vi "main_ctrl.vi"(8 "error in":errorcluster) -> (0 "error out":errorcluster caption="error")   [LabVIEW 2013]
uses:
  <vilib>/Rock Robotics/WPI/DriverStation/WPI_DriverStationRobotMode2.ctl
  typedefs/fg_typedef.ctl
  typedefs/vision enable.ctl
  typedefs/vision data.ctl
  typedefs/subStates.ctl
  typedefs/singleUseSubstate.ctl
  <vilib>/Rock Robotics/WPI/Solenoid/WPI_SolenoidValue.ctl
  <vilib>/Rock Robotics/WPI/Compressor/WPI_CompressorGetSetRefNum.vi
  <vilib>/Rock Robotics/WPI/RobotDrive/WPI_RobotDriveGetSetRefNum.vi
  <vilib>/Rock Robotics/WPI/RobotDrive/WPI_RobotDriveArcadeDrive_Standard(NoSaturation).vi
  <vilib>/Rock Robotics/WPI/Solenoid/WPI_SolenoidSetEnum.vi
panel:
  out "Robot Mode":T1
  out "Vision SPI":u32
  out "Vision IPS":dbl
  out "Main IPS":dbl
  out "Main SPI":u32
  # "MAIN CONTROL"
  # "holds robot control code - dual parallel state machine"
  # "SPI: milliseconds per iteration\nIPS: iterations per second"
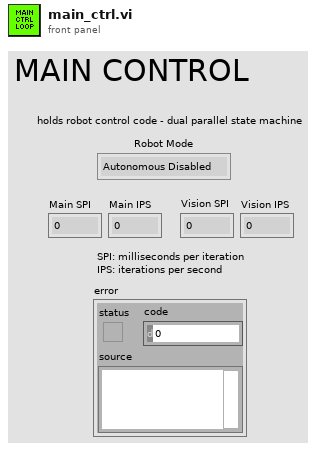
[diagram p1: front panel]
types:
  T1 = typedef "WPI_DriverStationRobotMode2.ctl" = enum16{"Autonomous Disabled", "Autonomous Enabled", "Teleop Disabled", "Teleop Enabled", "Timeout", "Finish", "Test Disabled", "Test Enabled"}
  T2 = typedef "vision data.ctl" = cluster{"x":dbl, "y":dbl, "area":dbl, "width":dbl, "height":dbl, "Hot Goal Present?":bool, "distance":dbl}
  T3 = typedef "vision enable.ctl" = enum16{"Enable", "Disable", "Stop"}
  T4 = typedef "fg_typedef.ctl" = enum16{"Get", "Set"}
  T5 = typedef "WPI_RobotDriveDevRef.ctl" = cluster{"DevStatus":errorcluster, "Motors[]":T6[], "Square Inputs":bool, "Max Output":dbl, "Isochronous":bool}
  T6 = typedef "WPI_MotorControlDeviceRef.ctl" = cluster{"DeviceStatus":errorcluster, "Type":enum16{"PWM", "CAN"}, "PWM":cluster{"Digital Module":T7, "PWM Channel":T8, "DeadBand":T9}, "CAN":cluster{"Device Number":u8, "Control Mode":T10, "Semaphore":T11, "Max Vout":dbl}, "Invert":bool, "TransformRef":T12, "InvTransformRef":T12}
  T7 = typedef "FPGA_TypedefDigitalModule.ctl" = enum16{"Digital Module 1", "Digital Module 2"}
  T8 = typedef "FPGA_DIOPWMChannel.ctl" = enum8{"PWM 1", "PWM 2", "PWM 3", "PWM 4", "PWM 5", "PWM 6", "PWM 7", "PWM 8", "PWM 9", "PWM 10", "Invalid"}
  T9 = typedef "WPI_PWMDeadband.ctl" = cluster{"Name":string, "maxPositivePwm":i32, "minPositivePwm":i32, "centerPwm":i32, "maxNegativePwm":i32, "minNegativePwm":i32, "angularRange":u16}
  T10 = typedef "WPI_CANJaguar_ControlMode.ctl" = enum8{"Percent VBus", "Current", "Speed", "Position", "Voltage"}
  T11 = typedef "Semaphore RefNum" = refnum<k1>
  T12 = typedef "WPI_PWMTransform_ConPane.ctl" = refnum<vi>
  T13 = typedef "WPI_CompressorDevRef.ctl" = cluster{"DevStatus":errorcluster, "DigitalInputDevRef":T14, "RelayDevRef":T16}
  T14 = typedef "WPI_DigitalInputDevRef.ctl" = cluster{"DevStatus":errorcluster, "DIO Channel":T15, "Digital Module":T7}
  T15 = typedef "FPGA_DIOChannel.ctl" = enum8{"DIO 1", "DIO 2", "DIO 3", "DIO 4", "DIO 5", "DIO 6", "DIO 7", "DIO 8", "DIO 9", "DIO 10", "DIO 11", "DIO 12", "DIO 13", "DIO 14", "Invalid"}
  T16 = typedef "WPI_RelayDevRef.ctl" = cluster{"DevStatus":errorcluster, "Relay Channel":T17, "Digital Module":T7, "Relay Direction":T18}
  T17 = typedef "FPGA_DIORelayChannel.ctl" = enum8{"Relay 1", "Relay 2", "Relay 3", "Relay 4", "Relay 5", "Relay 6", "Relay 7", "Relay 8", "Invalid"}
  T18 = typedef "WPI_RelayDirection.ctl" = enum16{"Both directions", "Forward only", "Reverse only"}
  T19 = typedef "WPI_CameraDevRef.ctl" = cluster{"Camera Address":string, "CameraStatus":errorcluster, "Acquire Image Notifier":refnum<notifier>}
  T20 = typedef "WPI_SolenoidDevRef.ctl" = cluster{"DevStatus":errorcluster, "Solenoid Module":T21, "Forward Solenoid Channel":T22, "Reverse Solenoid Channel":T22}
  T21 = typedef "FPGA_TypedefSolenoidModule.ctl" = enum16{"Solenoid Module 1", "Solenoid Module 2"}
  T22 = typedef "WPI_SolenoidChannel.ctl" = enum8{"Solenoid 1", "Solenoid 2", "Solenoid 3", "Solenoid 4", "Solenoid 5", "Solenoid 6", "Solenoid 7", "Solenoid 8", "Invalid"}
  T23 = typedef "IMAQ Image.ctl" = refnum<image>
  T24 = typedef "WPI_SolenoidValue.ctl" = enum16{"Off", "On", "Forward", "Reverse"}
  T25 = typedef "singleUseSubstate.ctl" = enum16{"null", "wait", "shift high", "shift low"}
  T26 = typedef "WPI_DriverStationDerivedRobotMode.ctl" = enum16{"Init", "Execute", "Stop"}
  T27 = typedef "subStates.ctl" = enum16{"null", "wait", "driver control", "auto", "manual override", "hold position", "rotate", "pickup", "pass", "load", "cock", "goto shoot", "shoot", "end"}
  T28 = typedef "Loop 2 Datatype.ctl" = cluster{"State":T27, "Waiting Loop":i32, "State to Wait For":i32, "Loop ID":i32, "Exit Value":i32, "Joystick":dbl}
  T29 = typedef "Loop 1 Datatype.ctl" = cluster{"State":T27, "Waiting Loop":i32, "State to Wait For":i32, "Loop ID":i32, "Exit Value":i32, "Joystick":dbl, "Index Up":bool, "Index Down":bool}
  T30 = typedef "Loop 3 Datatype.ctl" = cluster{"State":T27, "Waiting Loop":i32, "State to Wait For":i32, "Loop ID":i32, "Exit Value":i32, "Joystick":dbl, "Z Axis":dbl}
  T31 = typedef "Loop 0 Datatype.ctl" = cluster{"State":T27, "Waiting Loop":i32, "State to Wait For":i32, "Loop ID":i32, "Exit Value":i32, "X Axis":dbl, "Y Axis":dbl, "Z Axis":dbl}
  T32 = typedef "Loop 4 Datatype.ctl" = cluster{"State":T27, "Waiting Loop":i32, "State to Wait For":i32, "Loop ID":i32, "Exit Value":i32, "Joystick":dbl}
  T33 = cluster{"Vision mSPI":u32, "Main mSPI":u32, "Dash mSPI":u32}
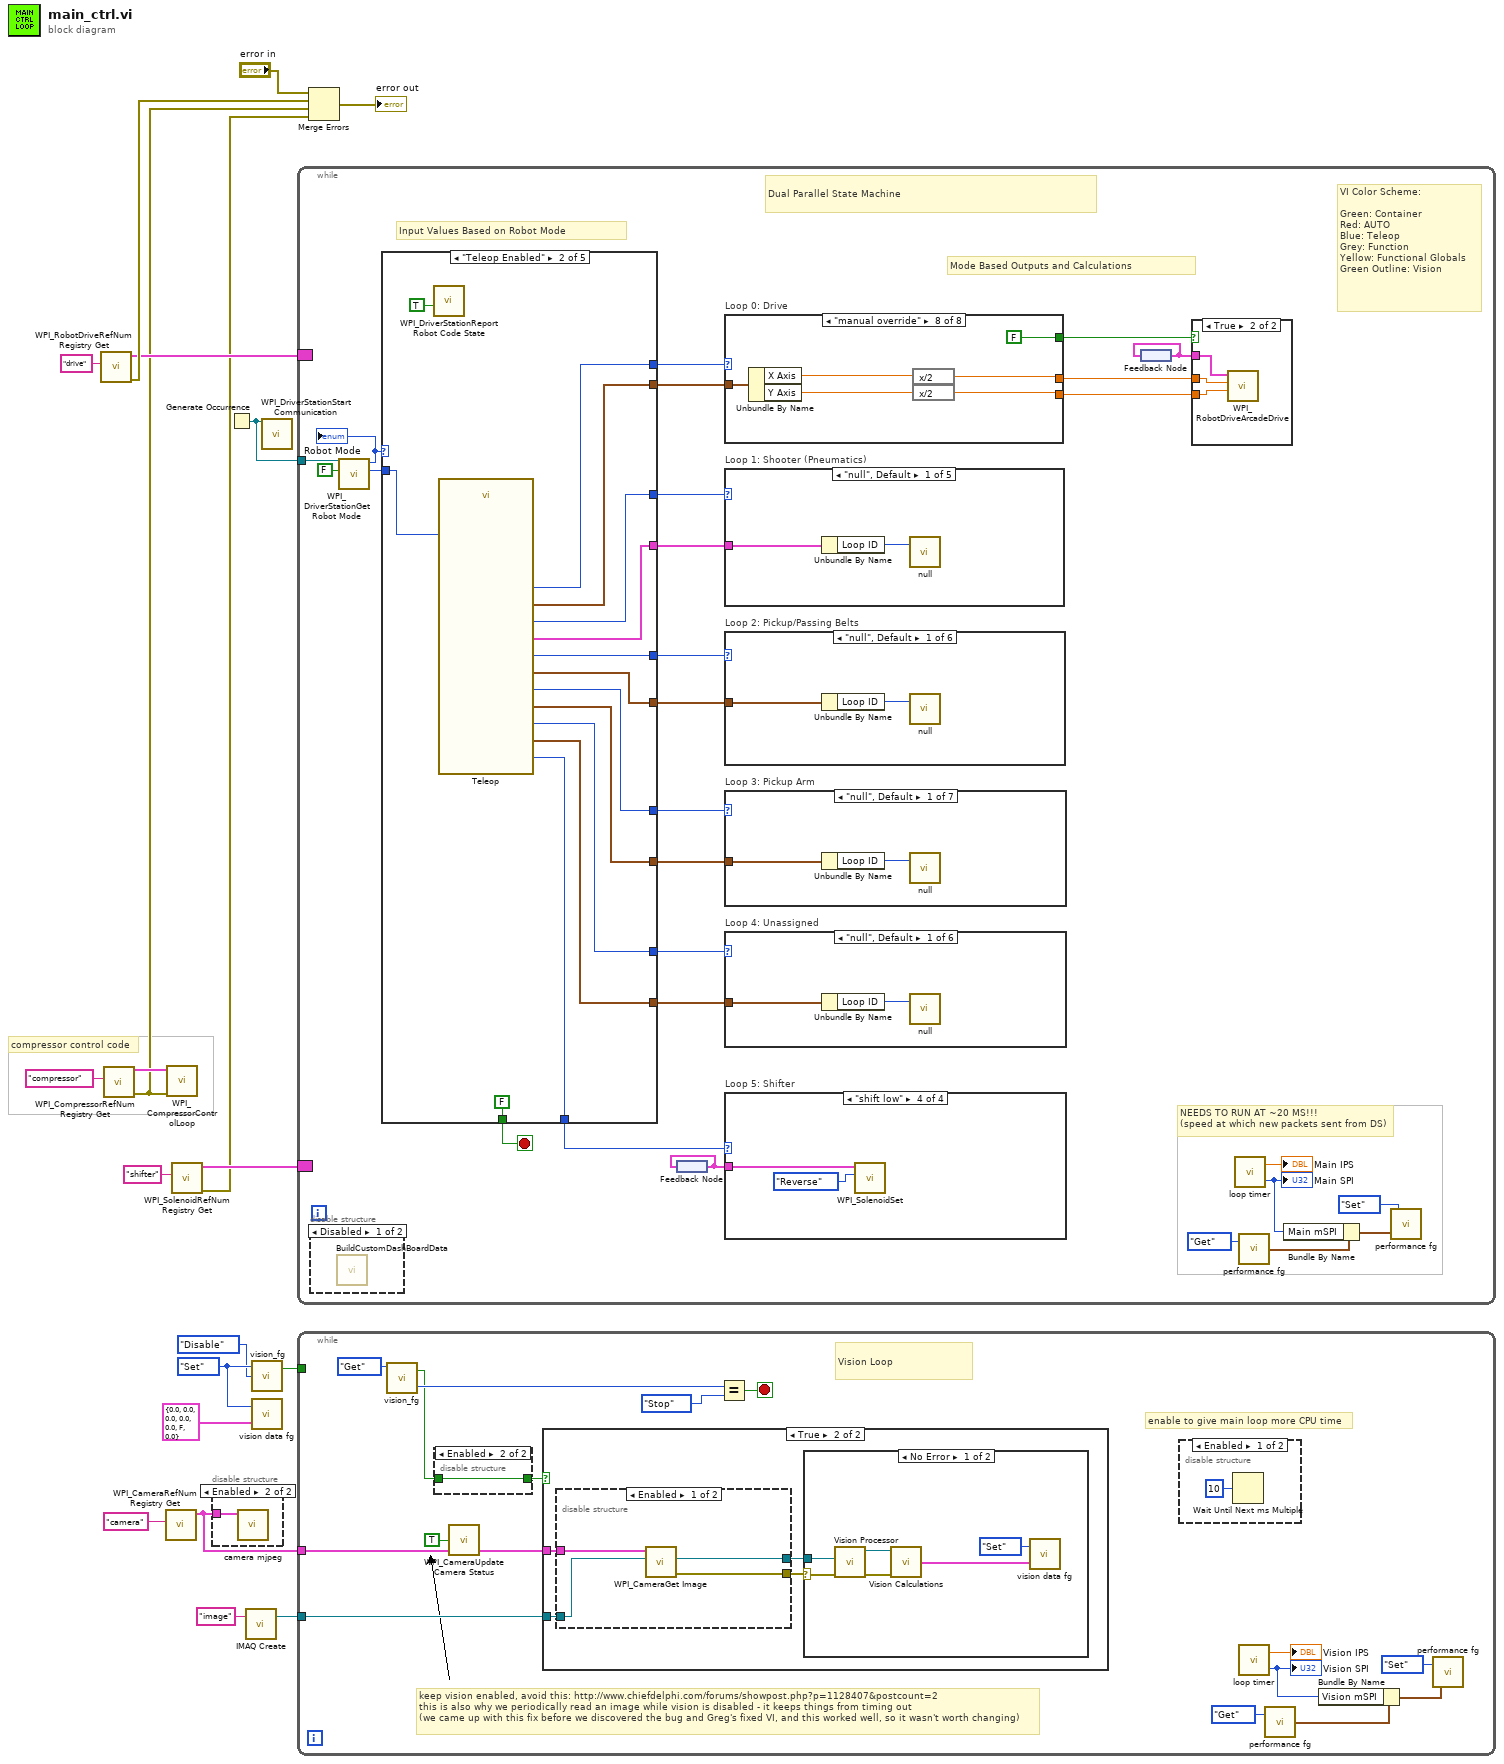
[diagram p0: block diagram]
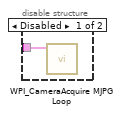
[diagram p2: hidden frame]
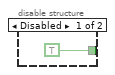
[diagram p3: hidden frame]
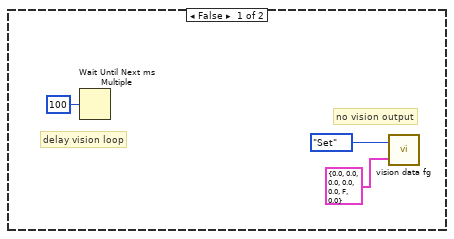
[diagram p5: hidden frame]
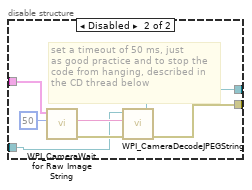
[diagram p7: hidden frame]
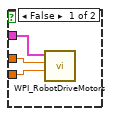
[diagram p9: hidden frame]
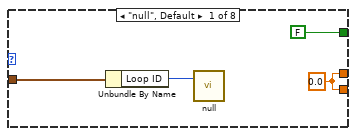
[diagram p10: hidden frame]
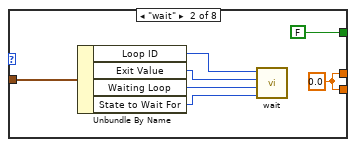
[diagram p11: hidden frame]
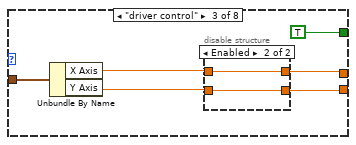
[diagram p12: hidden frame]
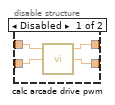
[diagram p13: hidden frame]
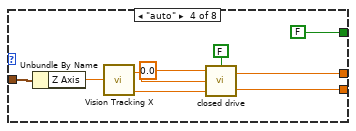
[diagram p14: hidden frame]
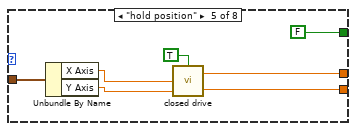
[diagram p15: hidden frame]
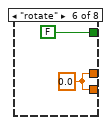
[diagram p16: hidden frame]
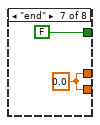
[diagram p17: hidden frame]
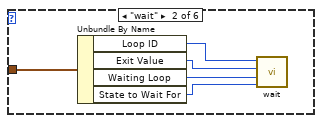
[diagram p18: hidden frame]
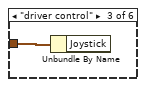
[diagram p19: hidden frame]
diagram:
  w7 = fg_typedef."Set" ("Enum")
  # "compressor control code"
  n1 = call <vilib>:"WPI_RobotDriveRefNum Registry Get.vi"("refnum name"="drive") -> ("error out"=w17:errorcluster, "RobotDriveDevRef"=w15:T5)  [unwired: 9 in]
  n2 = call <vilib>:"WPI_CompressorRefNum Registry Get.vi"("refnum name"="compressor") -> ("error out"=w10:errorcluster, "CompressorDevRef"=w14:T13)  [unwired: 9 in]
  n3 = call <vilib>:"WPI_CameraRefNum Registry Get.vi"("refnum name"="camera") -> ("CameraDevRef"=w4:T19)  [unwired: 9 in, 1 out]
  n4 = call <vilib>:"WPI_CompressorControlLoop.vi"("error in (no error)"=w10, "CompressorDevRef"=w14) -> ()  [unwired: 10 in]
  n5 = call <vilib>:"WPI_SolenoidRefNum Registry Get.vi"("refnum name"="shifter") -> ("error out"=w11:errorcluster, "SolenoidDevRef"=w13:T20)  [unwired: 9 in]
  n6 = disable-structure shown="Enabled" {
    disable-tunnel: w4 -> [w21 w22]
    frame Disabled {
      n7 = call <vilib>:"WPI_CameraAcquire MJPG Loop.vi"("CameraDevRef"=w21) -> ()  [unwired: 11 in]
    }
    frame Enabled {
      n8 = call "camera mjpeg.vi"("CameraDevRef"=w22) -> ()  [unwired: 11 in]
    }
  }
  n9 = Generate Occurrence() -> (w2:refnum<k4>)
  n10 = call "IMAQ Create"("Image Name"="image") -> ("New Image"=w9:T23)  [unwired: 4 in, 1 out]
  n11 = call "vision_fg.vi"("Action"=vision_enable."Disable", "Menu"=w7) -> ("Enabled?"=w8:bool)  [unwired: 1 in, 1 out]
  n12 = call "vision data fg.vi"("Input"=T2 {"x"=0.0, "y"=0.0, "area"=0.0, "width"=0.0, "height"=0.0, "Hot Goal Present?"=FALSE, "distance"=0.0} ("Cluster"), "Menu"=w7) -> ()  [unwired: 1 out]
  n13 = call <vilib>:"WPI_DriverStationStart Communication.vi"("occurrence"=w2) -> ()  [unwired: 11 in]
  n14 = while {
    tunnel: w2 -> [w25]
    border: w15 -> [_]
    border: w13 -> [_]
    stop <- w46 stop-if-true
    # "VI Color Scheme:\n\nGreen: Container\nRed: AUTO\nBlue: Teleop\nGrey: Function\nYellow: Functional Globals\nGreen Outline: Vision"
    # "Input Values Based on Robot Mode"
    # "Mode Based Outputs and Calculations"
    # "NEEDS TO RUN AT ~20 MS!!!\n(speed at which new packets sent from DS)"
    # "Dual Parallel State Machine"
    n15 = disable-structure shown="Disabled" {
      frame Disabled {
        n16 = call "BuildCustomDashBoardData.vi"() -> ()  [unwired: 12 in]
      }
      frame Enabled {
      }
    }
    n17 = call <vilib>:"WPI_DriverStationGet Robot Mode.vi"("Finish"=FALSE, "DS Occurrence"=w25) -> ("Call Context"=w24:T26, "Robot Mode"=w23:T1)  [unwired: 8 out]
    "Robot Mode" <- w23
    n18 = case shown="\"Teleop Enabled\"" w23 {
      tunnel: [w155 w172 w174 w180 w186] -> w27
      tunnel: w24 -> [w146 w168 _ _ _]
      tunnel: [w153 w171 w174 w180 w186] -> w48
      tunnel: [w147 w169 singleUseSubstate."null" ("SubState 5") singleUseSubstate."null" ("SubState 5") singleUseSubstate."null" ("SubState 5")] -> w47
      tunnel: [FALSE FALSE FALSE FALSE TRUE] -> w46
      tunnel: [w157 w167 w174 w180 w186] -> w39
      tunnel: [w156 w166 _ _ _] -> w40
      tunnel: [w154 w165 _ _ _] -> w38
      tunnel: [w152 w164 _ _ _] -> w37
      tunnel: [w150 w163 _ _ _] -> w35
      tunnel: [w148 w162 _ _ _] -> w34
      tunnel: [w149 w161 w174 w180 w186] -> w33
      tunnel: [w151 w160 w174 w180 w186] -> w32
      frame "Autonomous Enabled" {
        n19 = call <vilib>:"WPI_DriverStationReport Robot Code State.vi"("Autonomous"=TRUE) -> ()  [unwired: 10 in, 1 out]
        n20 = call "Autonomous.vi"("Call Context"=w146) -> ("SubState 2"=w153:T27, "Loop 2 Data"=w152:T28, "SubState 1"=w155:T27, "Loop 1 Data"=w154:T29, "Loop 3 Data"=w150:T30, "SubState 0"=w157:T27, "SubState 3"=w151:T27, "Loop 0 Data"=w156:T31, "Loop 4 Data"=w148:T32, "SubState 4"=w149:T27, "SubState 5"=w147:T25)
      }
      frame "Teleop Enabled" {
        n21 = call <vilib>:"WPI_DriverStationReport Robot Code State.vi"("TeleOp"=TRUE) -> ()  [unwired: 10 in, 1 out]
        n22 = call "Teleop.vi"("Call Context"=w168) -> ("SubState 3"=w160:T27, "SubState 4"=w161:T27, "SubState 5"=w169:T25, "Loop 3 Data"=w163:T30, "Loop 4 Data"=w162:T32, "SubState 0"=w167:T27, "Loop 1 Data"=w165:T29, "Loop 0 Data"=w166:T31, "SubState 1"=w172:T27, "Loop 2 Data"=w164:T28, "SubState 2"=w171:T27)  [unwired: 8 in]
      }
      frame "Autonomous Disabled", "Teleop Disabled", "Timeout" {
        w174 = subStates."null" ("SubState 0")
        # "set all loops to null"
        # "make sure to disable vision\nwe don't need it here"
        # "robot disabled, timeout"
        n23 = call <vilib>:"WPI_DriverStationReport Robot Code State.vi"("Disabled"=TRUE) -> ()  [unwired: 10 in, 1 out]
        n24 = call "vision_fg.vi"("Action"=vision_enable."Disable", "Menu"=fg_typedef."Set") -> ()  [unwired: 1 in, 2 out]
      }
      frame "Test Disabled", "Test Enabled" {
        w180 = subStates."null" ("SubState 0")
        # "set all loops to null"
        # "make sure to disable vision\nwe don't need it here"
        # "test, unused"
        n25 = call <vilib>:"WPI_DriverStationReport Robot Code State.vi"("Test"=TRUE) -> ()  [unwired: 10 in, 1 out]
        n26 = call "vision_fg.vi"("Action"=vision_enable."Disable", "Menu"=fg_typedef."Set") -> ()  [unwired: 1 in, 2 out]
      }
      frame "Finish" {
        w186 = subStates."end"  # Stop All Loops
        # "stop the while loop"
        # "stop DS comms"
        # "stop vision loop"
        n27 = call <vilib>:"WPI_DriverStationStop Communication.vi"("StopCommunication"=TRUE) -> ()  [unwired: 10 in, 1 out]
        n28 = call "vision_fg.vi"("Action"=vision_enable."Stop", "Menu"=fg_typedef."Set") -> ()  [unwired: 1 in, 2 out]
      }
    }
    n29 = feedback #1() -> (w36:T20)
    n30 = feedback-in #1(w36) -> ()
    n31 = case "Loop 0: Drive" shown="\"manual override\"" w39 {
      tunnel: w40 -> [w58 w62 w72 w81 w93 _ _ w104]
      tunnel: [w56 w60 w68 w86 w90 w96 w98 w100] -> w30
      tunnel: [w56 w60 w67 w85 w89 w96 w98 w99] -> w29
      tunnel: [FALSE FALSE TRUE FALSE FALSE FALSE FALSE FALSE] -> w31
      frame "null", Default {
        w56 = 0.0 ("X Axis")
        n32 = Unbundle By Name(w58) -> ("Loop ID"=w59:i32)
        n33 = call "null.vi"("This Loop ID"=w59) -> ()  [unwired: 2 in]
      }
      frame "wait" {
        w60 = 0.0 ("X Axis")
        n34 = Unbundle By Name(w62) -> ("Loop ID"=w66:i32, "Exit Value"=w65:i32, "Waiting Loop"=w64:i32, "State to Wait For"=w63:i32)
        n35 = call "wait.vi"("State to wait for"=w63, "Waiting Loop ID"=w64, "time (ms)"=w65, "Current Loop ID"=w66) -> ()  [unwired: 1 out]
      }
      frame "driver control" {
        n36 = Unbundle By Name(w72) -> ("X Axis"=w70:dbl, "Y Axis"=w69:dbl)
        n37 = disable-structure shown="Enabled" {
          disable-tunnel: w70 -> [w76 w78]
          disable-tunnel: w69 -> [w75 w77]
          disable-tunnel: [w74 w78] -> w68
          disable-tunnel: [w73 w77] -> w67
          frame Disabled {
            n38 = call "calc arcade drive pwm.vi"("Y axis value"=w75, "X axis value"=w76) -> ("Right Speed"=w73:dbl, "Left Speed"=w74:dbl)  [unwired: 1 in, 1 out]
          }
          frame Enabled {
          }
        }
      }
      frame "auto" {
        n39 = Unbundle By Name(w81) -> ("Z Axis"=w80:dbl)
        n40 = call "Vision Tracking X.vi"("Tweak"=w80) -> ("right speed"=w79:dbl, "left speed"=w83:dbl)
        n41 = call "closed drive.vi"("Acrade Drive?"=FALSE, "Y axis value (Left)"=w83, "X axis value (Right)"=w79, "Threshold (.4)"=0.0 ("Threshold")) -> ("right"=w85:dbl, "left"=w86:dbl)
      }
      frame "hold position" {
        n42 = Unbundle By Name(w93) -> ("X Axis"=w92:dbl, "Y Axis"=w91:dbl)
        n43 = call "closed drive.vi"("Acrade Drive?"=TRUE, "Y axis value (Left)"=w91, "X axis value (Right)"=w92) -> ("right"=w89:dbl, "left"=w90:dbl)  [unwired: 1 in]
      }
      frame "rotate" {
        w96 = 0.0 ("X Axis")
      }
      frame "end" {
        w98 = 0.0 ("X Axis")
      }
      frame "manual override" {
        n44 = Unbundle By Name(w104) -> ("X Axis"=w103:dbl, "Y Axis"=w102:dbl)
        n45 = expression code="x/2"(w103) -> (w100:dbl)
        n46 = expression code="x/2"(w102) -> (w99:dbl)
      }
    }
    n47 = case "Loop 1: Shooter (Pneumatics)" shown="\"null\", Default" w27 {
      tunnel: w38 -> [w137 w139 _ _ w144]
      frame "null", Default {
        n48 = Unbundle By Name(w137) -> ("Loop ID"=w138:i32)
        n49 = call "null.vi"("This Loop ID"=w138) -> ()  [unwired: 2 in]
      }
      frame "wait" {
        n50 = Unbundle By Name(w139) -> ("Loop ID"=w143:i32, "Exit Value"=w142:i32, "Waiting Loop"=w141:i32, "State to Wait For"=w140:i32)
        n51 = call "wait.vi"("State to wait for"=w140, "Waiting Loop ID"=w141, "time (ms)"=w142, "Current Loop ID"=w143) -> ()  [unwired: 1 out]
      }
      frame "driver control" {
      }
      frame "auto" {
      }
      frame "manual override" {
        n52 = Unbundle By Name(w144) -> ()  [unwired: 1 out]
      }
    }
    n53 = case "Loop 2: Pickup/Passing Belts" shown="\"null\", Default" w48 {
      tunnel: w37 -> [w130 w131 _ _ w136 _]
      frame "null", Default {
        n54 = Unbundle By Name(w130) -> ("Loop ID"=w129:i32)
        n55 = call "null.vi"("This Loop ID"=w129) -> ()  [unwired: 2 in]
      }
      frame "wait" {
        n56 = Unbundle By Name(w131) -> ("Loop ID"=w135:i32, "Exit Value"=w134:i32, "Waiting Loop"=w133:i32, "State to Wait For"=w132:i32)
        n57 = call "wait.vi"("State to wait for"=w132, "Waiting Loop ID"=w133, "time (ms)"=w134, "Current Loop ID"=w135) -> ()  [unwired: 1 out]
      }
      frame "driver control" {
      }
      frame "auto" {
      }
      frame "manual override" {
        n58 = Unbundle By Name(w136) -> ()  [unwired: 1 out]
      }
      frame "pickup" {
      }
    }
    n59 = case "Loop 3: Pickup Arm" shown="\"null\", Default" w32 {
      tunnel: w35 -> [w115 w116 w121 _ w122 w123 w124]
      frame "null", Default {
        n60 = Unbundle By Name(w115) -> ("Loop ID"=w114:i32)
        n61 = call "null.vi"("This Loop ID"=w114) -> ()  [unwired: 2 in]
      }
      frame "wait" {
        n62 = Unbundle By Name(w116) -> ("Loop ID"=w120:i32, "Exit Value"=w119:i32, "Waiting Loop"=w118:i32, "State to Wait For"=w117:i32)
        n63 = call "wait.vi"("State to wait for"=w117, "Waiting Loop ID"=w118, "time (ms)"=w119, "Current Loop ID"=w120) -> ()  [unwired: 1 out]
      }
      frame "driver control" {
        n64 = Unbundle By Name(w121) -> ()  [unwired: 1 out]
      }
      frame "auto" {
      }
      frame "manual override" {
        n65 = Unbundle By Name(w122) -> ()  [unwired: 1 out]
      }
      frame "pickup" {
        n66 = Unbundle By Name(w123) -> ()  [unwired: 1 out]
      }
      frame "shoot" {
        n67 = Unbundle By Name(w124) -> ()  [unwired: 1 out]
      }
    }
    n68 = case "Loop 4: Unassigned" shown="\"null\", Default" w33 {
      tunnel: w34 -> [w106 w107 w112 _ w113 _]
      frame "null", Default {
        n69 = Unbundle By Name(w106) -> ("Loop ID"=w105:i32)
        n70 = call "null.vi"("This Loop ID"=w105) -> ()  [unwired: 2 in]
      }
      frame "wait" {
        n71 = Unbundle By Name(w107) -> ("Loop ID"=w111:i32, "Exit Value"=w110:i32, "Waiting Loop"=w109:i32, "State to Wait For"=w108:i32)
        n72 = call "wait.vi"("State to wait for"=w108, "Waiting Loop ID"=w109, "time (ms)"=w110, "Current Loop ID"=w111) -> ()  [unwired: 1 out]
      }
      frame "driver control" {
        n73 = Unbundle By Name(w112) -> ()  [unwired: 1 out]
      }
      frame "auto" {
      }
      frame "manual override" {
        n74 = Unbundle By Name(w113) -> ()  [unwired: 1 out]
      }
      frame "pickup" {
      }
    }
    n75 = case "Loop 5: Shifter" shown="\"shift low\"" w47 {
      tunnel: w36 -> [_ _ w126 w127]
      frame "null", Default {
      }
      frame "wait" {
      }
      frame "shift high" {
        n76 = call-poly <vilib>:"WPI_SolenoidSet.vi"("Value"=WPI_SolenoidValue."Forward", "SolenoidDevRef"=w126) -> ()  [unwired: 8 in, 2 out]
      }
      frame "shift low" {
        n77 = call-poly <vilib>:"WPI_SolenoidSet.vi"("Value"=WPI_SolenoidValue."Reverse", "SolenoidDevRef"=w127) -> ()  [unwired: 8 in, 2 out]
      }
    }
    n78 = feedback #2() -> (w28:T5)
    n79 = feedback-in #2(w28) -> ()
    n80 = case shown="True" w31 {
      tunnel: w30 -> [w51 w55]
      tunnel: w29 -> [w50 w54]
      tunnel: w28 -> [w52 w53]
      frame False {
        n81 = call <vilib>:"WPI_RobotDriveMotors.vi"("RightSpeed"=w50, "LeftSpeed"=w51, "RobotDriveDevRef"=w52) -> ()  [unwired: 6 in, 3 out]
      }
      frame True {
        n82 = call-poly <vilib>:"WPI_RobotDriveArcadeDrive.vi"("Y axis value"=w54, "X axis value"=w55, "RobotDriveDevRef"=w53) -> ()  [unwired: 6 in, 3 out]
      }
    }
    n83 = call "loop timer.vi"() -> ("IPS"=→"Main IPS":dbl, "SPI"=w45:u32)  [unwired: 1 in]
    "Main SPI" <- w45
    n84 = call "performance fg.vi"("Menu"=fg_typedef."Get") -> ("Output"=w42:T33)  [unwired: 1 in]
    n85 = Bundle By Name(cluster=w42, "Main mSPI"=w45) -> (w41:T33)
    n86 = call "performance fg.vi"("Input"=w41, "Menu"=fg_typedef."Set") -> ()  [unwired: 1 out]
  }
  n87 = while {
    tunnel: w9 -> [w205]
    tunnel: w4 -> [w204]
    tunnel: w8 -> [_]
    stop <- w206 stop-if-true
    # "keep vision enabled, avoid this: http://www.chiefdelphi.com/forums/showpost.php?p=1128407&postcount=2\nthis is also why we periodically read an image while vision is disabled - it keeps things from timing out\n(we came up with this fix before we discovered the bug and Greg's fixed VI, and this worked well, so it wasn't worth changing)"
    # "enable to give main loop more CPU time"
    # "Vision Loop"
    n88 = call "vision_fg.vi"("Menu"=fg_typedef."Get" ("Enum")) -> ("State Out"=w200:T3, "Enabled?"=w191:bool)  [unwired: 2 in]
    n89 = disable-structure shown="Enabled" {
      disable-tunnel: [TRUE w208] -> w192
      disable-tunnel: w191 -> [_ w208]
      frame Disabled {
      }
      frame Enabled {
      }
    }
    n90 = call <vilib>:"WPI_CameraUpdate Camera Status.vi"("CameraDevRef In"=w204, "Enable Vision"=TRUE) -> ("CameraDevRef Out"=w203:T19)  [unwired: 3 in]
    n91 = case shown="True" w192 {
      tunnel: w205 -> [_ w216]
      tunnel: w203 -> [_ w215]
      frame False {
        # "no vision output"
        # "delay vision loop"
        n92 = Wait Until Next ms Multiple(millisecond multiple=u32 100) -> ()  [unwired: 1 out]
        n93 = call "vision data fg.vi"("Input"=T2 {"x"=0.0, "y"=0.0, "area"=0.0, "width"=0.0, "height"=0.0, "Hot Goal Present?"=FALSE, "distance"=0.0} ("Cluster"), "Menu"=fg_typedef."Set" ("Enum")) -> ()  [unwired: 1 out]
      }
      frame True {
        n94 = disable-structure shown="Enabled" {
          disable-tunnel: w216 -> [w225 w229]
          disable-tunnel: w215 -> [w226 w231]
          disable-tunnel: [w224 w228] -> w214
          disable-tunnel: [w223 w227] -> w213
          frame Enabled {
            n95 = call <vilib>:"WPI_CameraGet Image.vi"("Image"=w225, "CameraDevRef"=w226) -> ("error out"=w223:errorcluster, "Image Out"=w224:T23)  [unwired: 7 in, 1 out]
          }
          frame Disabled {
            # "set a timeout of 50 ms, just\nas good practice and to stop the \ncode from hanging, described in \nthe CD thread below"
            n96 = call <vilib>:"WPI_CameraWait for Raw Image String.vi"("Timeout in ms (-1)"=50, "CameraDevRef"=w231) -> ("error out"=w233:errorcluster, "String"=w232:string)  [unwired: 3 in, 5 out]
            n97 = call <vilib>:"WPI_CameraDecodeJPEGString.vi"("error in"=w233, "Compressed Image"=w232, "Image In"=w229) -> ("error out"=w227:errorcluster, "Image Out"=w228:T23)  [unwired: 3 out]
          }
        }
        n98 = case shown="No Error" w213 {
          selector: w213 -> [w221 _]
          tunnel: w214 -> [w220 _]
          frame No Error {
            n99 = call "Vision Processor.vi"("error in"=w221, "Image In"=w220) -> ("error out"=w218:errorcluster, "Image Out"=w219:T23)  [unwired: 5 in]
            n100 = call "Vision Calculations.vi"("Image In"=w219, "error in"=w218) -> ("Vision Data"=w217:T2)  [unwired: 3 in]
            n101 = call "vision data fg.vi"("Input"=w217, "Menu"=fg_typedef."Set" ("Enum")) -> ()  [unwired: 1 out]
          }
          frame Error {
          }
        }
      }
    }
    n102 = Equal?(x=w200, y=vision_enable."Stop") -> (x = y?=w206:bool)
    n103 = disable-structure shown="Enabled" {
      frame Enabled {
        n104 = Wait Until Next ms Multiple(millisecond multiple=u32 10) -> ()  [unwired: 1 out]
      }
      frame Disabled {
      }
    }
    n105 = call "loop timer.vi"() -> ("IPS"=→"Vision IPS":dbl, "SPI"=w198:u32)  [unwired: 1 in]
    "Vision SPI" <- w198
    n106 = call "performance fg.vi"("Menu"=fg_typedef."Get") -> ("Output"=w196:T33)  [unwired: 1 in]
    n107 = Bundle By Name(cluster=w196, "Vision mSPI"=w198) -> (w195:T33)
    n108 = call "performance fg.vi"("Input"=w195, "Menu"=fg_typedef."Set") -> ()  [unwired: 1 out]
  }
  n109 = Merge Errors("error in", w17, w10, w11) -> (→"error out":errorcluster)
